vi "Total Transfered Energy from Exposed Saline Water.vi"(4 "Adde Vapor":dbl[unit], 5 "Salinity Evaporator Water OUT":dbl=0.004, 6 "Salinity Evaporator Water IN":dbl=0.0035, 7 "Temp Evap Water OUT":dbl[unit], 8 "Temp Evap Water IN":dbl[unit]) -> (0 "S1 is greater Than S2\nThat is Wrong":bool, 1 "Total Transfered Energy from Exposed Saline Water":dbl[unit], 2 "Mass FLow Rate of \nOutput Expose Saline Water":dbl[unit], 3 "Mass FLow Rate of \nInput Expose Saline Water":dbl[unit])   [LabVIEW 2018]
panel:
  out "Total Enthalphy of \nOut Put Exposed Saline Water":dbl[unit]
  out "Total Enthalphy of In Put Exposed Saline Water":dbl[unit]
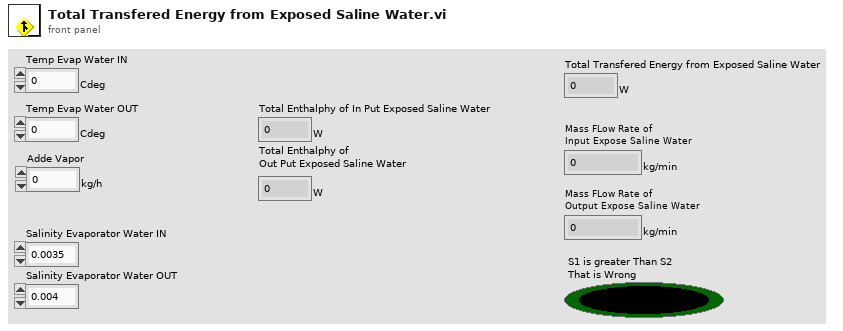
[diagram p1: front panel]
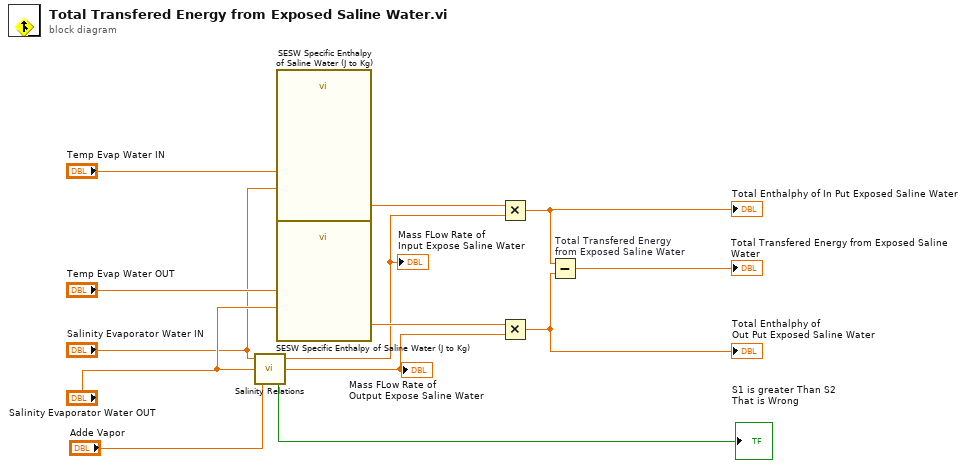
[diagram p0: block diagram]
diagram:
  n1 = call "Salinity Relations.vi"("Adde Vapor"="Adde Vapor", "S2 / Salinity of Output Exposed Saline Water"="Salinity Evaporator Water OUT", "S1 / Salinity of Input Exposed Saline Water"="Salinity Evaporator Water IN") -> ("S1 is greater Than S2\nThat is Wrong"=→"S1 is greater Than S2\nThat is Wrong":bool, "Output Exposed Saline Water"=w6:dbl[unit], "Input Exposed Saline Water"=w7:dbl[unit])
  "Mass FLow Rate of \nOutput Expose Saline Water" <- w6
  "Mass FLow Rate of \nInput Expose Saline Water" <- w7
  n2 = call "SESW Specific Enthalpy of Saline Water (J to Kg).vi"("Salinity"="Salinity Evaporator Water IN", "Sailne Water Temprature"="Temp Evap Water IN") -> ("SESW"=w12:dbl[unit])
  n3 = call "SESW Specific Enthalpy of Saline Water (J to Kg).vi"("Salinity"="Salinity Evaporator Water OUT", "Sailne Water Temprature"="Temp Evap Water OUT") -> ("SESW"=w13:dbl[unit])
  n4 = Multiply(x=w12, y=w7) -> (x*y=w11:dbl[unit])
  "Total Enthalphy of In Put Exposed Saline Water" <- w11
  n5 = Multiply(x=w13, y=w6) -> (x*y=w10:dbl[unit])
  "Total Enthalphy of \nOut Put Exposed Saline Water" <- w10
  n6 = Subtract "Total Transfered Energy \nfrom Exposed Saline Water"(x=w11, y=w10) -> (x-y=→"Total Transfered Energy from Exposed Saline Water":dbl[unit])
